vi "Scott -- strain -- Ag controller.vi"(8 "error in (no error)":errorcluster, 10 "voltage IN":dbl, 11 "VISA resource name IN":refnum<visa-resource-name>) -> (0 "error out":errorcluster, 1 "No Errror!":bool, 2 "voltage OUT":dbl, 3 "VISA resource name OUT":refnum<visa-resource-name>)   [LabVIEW 2014]
uses:
  Q - not nan -- real.vi
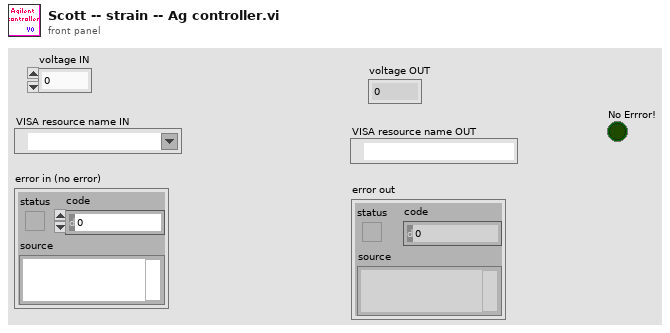
[diagram p1: front panel]
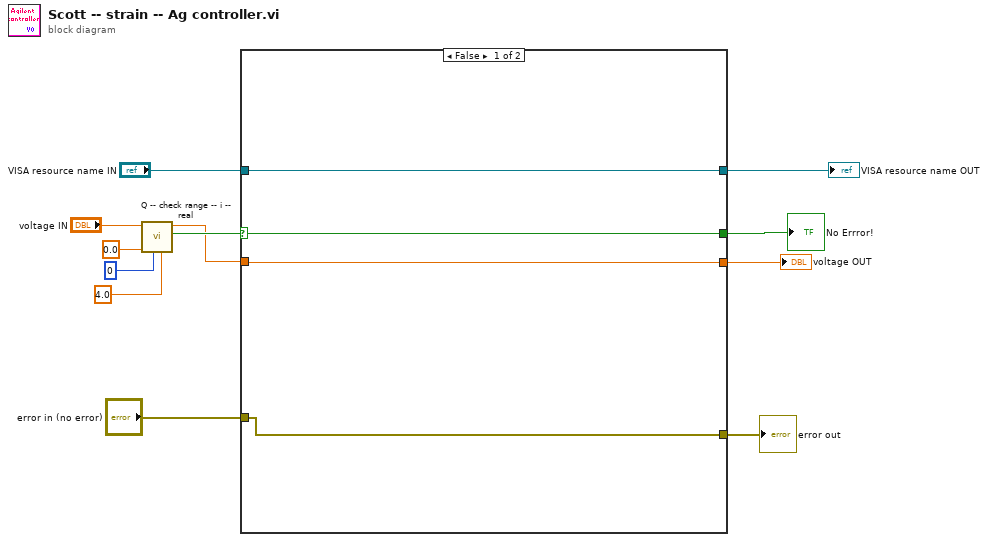
[diagram p0: block diagram]
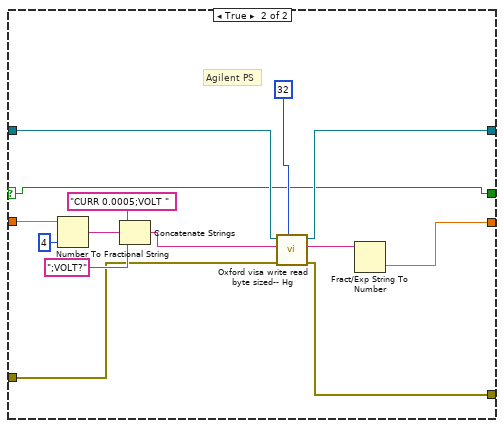
[diagram p2: hidden frame]
diagram:
  n1 = call "Q -- check range -- i -- real.vi"("upper"=4.0, "lower"=0, "default"=0.0, "number"="voltage IN") -> ("in range?"=w3:bool, "number in range"=w1:dbl)  [unwired: 5 in, 1 out]
  n2 = case shown="False" w3 {
    selector: w3 -> [w16 w17]
    tunnel: [w14 w26] -> w12
    tunnel: "VISA resource name IN" -> [w13 w23]
    tunnel: [w13 w22] -> w10
    tunnel: "error in (no error)" -> [w15 w20]
    tunnel: [w15 w19] -> w8
    tunnel: w1 -> [w14 w18]
    tunnel: [w16 w17] -> w2
    frame False {
    }
    frame True {
      # "Agilent PS"
      n3 = Number To Fractional String(number=w18, precision (6)=4) -> (F-format string=w30:string)  [unwired: 2 in]
      n4 = Concatenate Strings("CURR 0.0005;VOLT ", w30, ";VOLT?") -> (w25:string)
      n5 = call "Oxford visa write read byte sized-- Hg.vi"("byte count"=u32 32, "error in (no error)"=w20, "write buffer"=w25, "VISA resource name"=w23) -> ("error out"=w19:errorcluster, "read buffer"=w24:string, "VISA resource name out"=w22:refnum<visa-resource-name>)  [unwired: 5 in]
      n6 = Fract/Exp String To Number(string=w24) -> (number=w26:dbl)  [unwired: 3 in, 1 out]
    }
  }
  "voltage OUT" <- w12
  "VISA resource name OUT" <- w10
  "error out" <- w8
  "No Errror!" <- w2
